vi "Affichage - 2 cam - 2P.vi"(8 "Couleur rectangle":u32(colorbox)=16775680, 9 "Caméra D":T1, 10 "Choix cam":u16, 11 "Caméra G":T1) -> (2 "Image 2D":picture)   [LabVIEW 2013]
uses:
  <vilib>/picture/picture.llb/Draw True-Color Pixmap.vi
panel:
  in  "Couleur rectangle 2":u32(colorbox)=16775680
  # "Affichage"
  # "Pour un rectangle"
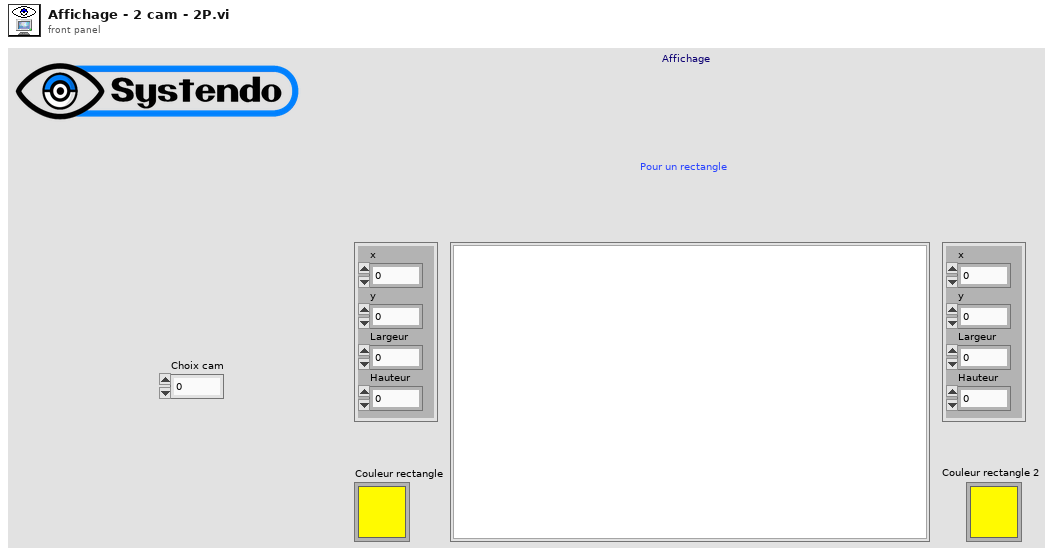
[diagram p1: front panel]
types:
  T1 = cluster{"x":i16, "y":i16, "Largeur":i16, "Hauteur":i16}
  T2 = typedef "imagedata.ctl" = cluster{"image type":i32, "image depth":i32, "image":u8[], "mask":u8[], "colors":u32[], "Rectangle":cluster{"left":i16, "top":i16, "right":i16, "bottom":i16}}
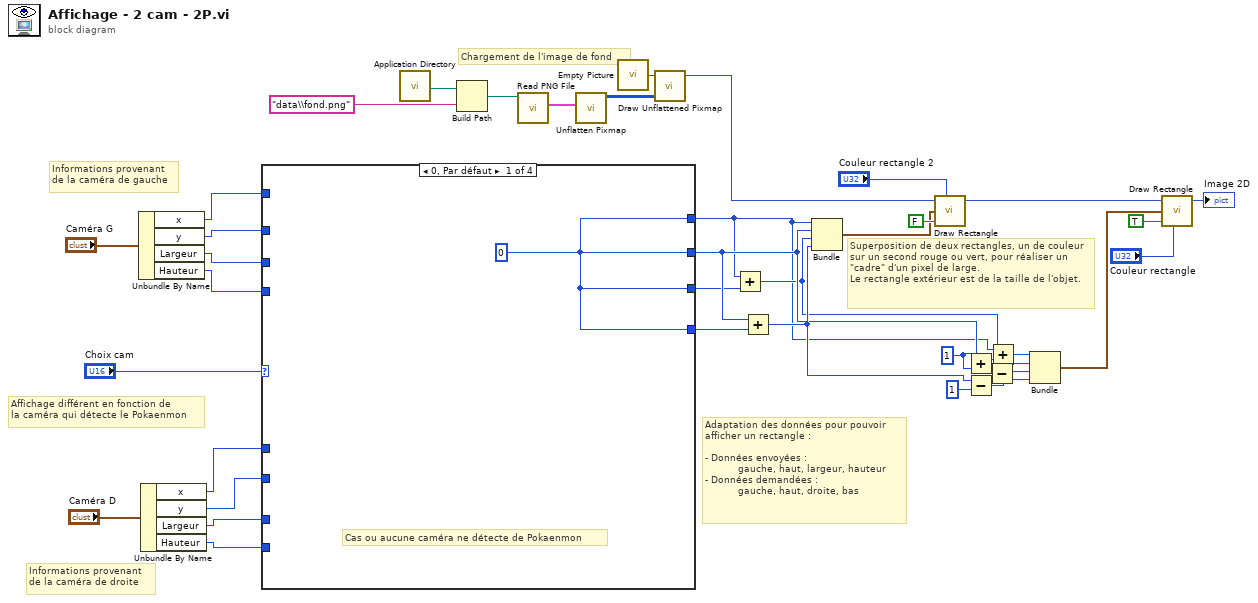
[diagram p0: block diagram]
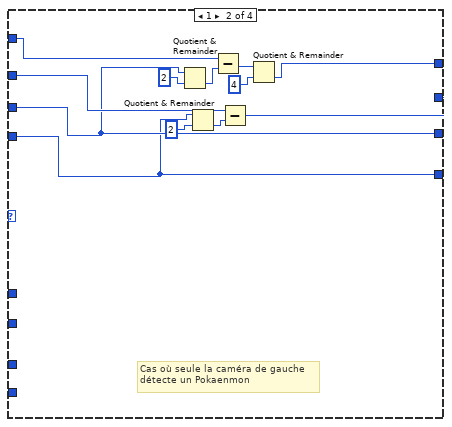
[diagram p2: hidden frame]
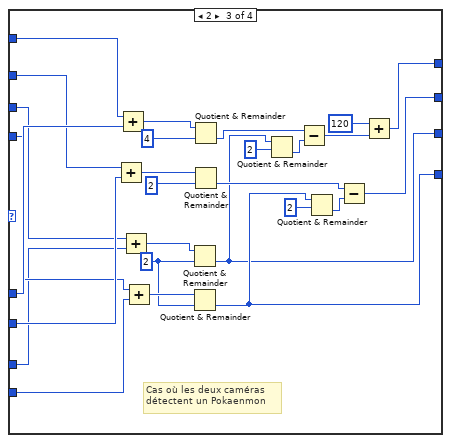
[diagram p3: hidden frame]
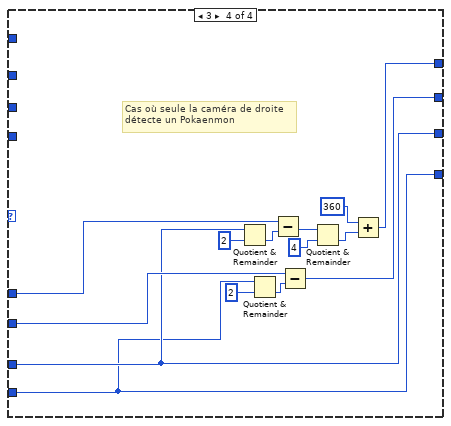
[diagram p4: hidden frame]
diagram:
  w15 = i16 1 ("y")
  w12 = i16 1 ("y")
  # "Chargement de l'image de fond"
  # "Superposition de deux rectangles, un de couleur sur un second rouge ou vert, pour réaliser un \"cadre\" d'un pixel de large.\nLe rectangle extérieur est de la taille de l'objet."
  # "Adaptation des données pour pouvoir\nafficher un rectangle :\n\n- Données envoyées :\n           gauche, haut, largeur, hauteur\n- Données demandées :\n           gauche, haut, droite, bas"
  # "Informations provenant\nde la caméra de droite"
  # "Informations provenant\nde la caméra de gauche"
  # "Affichage différent en fonction de\nla caméra qui détecte le Pokaenmon"
  n1 = Unbundle By Name("Caméra G") -> ("x"=w30:i16, "y"=w29:i16, "Largeur"=w28:i16, "Hauteur"=w27:i16)
  n2 = Unbundle By Name("Caméra D") -> ("x"=w23:i16, "y"=w24:i16, "Largeur"=w25:i16, "Hauteur"=w26:i16)
  n3 = case shown="0, Par défaut" "Choix cam" {
    tunnel: [w39 w43 w61 w88] -> w34
    tunnel: [w39 w49 w60 w90] -> w37
    tunnel: [w39 w47 w52 w83] -> w33
    tunnel: [w39 w41 w58 w80] -> w36
    tunnel: w23 -> [_ _ w71 w91]
    tunnel: w24 -> [_ _ w69 w92]
    tunnel: w25 -> [_ _ w66 w83]
    tunnel: w26 -> [_ _ w68 w80]
    tunnel: w27 -> [_ w41 w67 _]
    tunnel: w28 -> [_ w47 w65 _]
    tunnel: w29 -> [_ w50 w70 _]
    tunnel: w30 -> [_ w51 w72 _]
    frame 0, Default {
      w39 = 0
      # "Cas ou aucune caméra ne détecte de Pokaenmon"
    }
    frame 1 {
      # "Cas où seule la caméra de gauche\ndétecte un Pokaenmon"
      n4 = Quotient & Remainder(x=w47, y=u16 2) -> (floor(x/y)=w46:u16)  [unwired: 1 out]
      n5 = Quotient & Remainder(x=w41, y=u16 2) -> (floor(x/y)=w40:u16)  [unwired: 1 out]
      n6 = Subtract(x=w51, y=w46) -> (x-y=w44:u16)
      n7 = Subtract(x=w50, y=w40) -> (x-y=w49:u16)
      n8 = Quotient & Remainder(x=w44, y=u16 4) -> (floor(x/y)=w43:u16)  [unwired: 1 out]
    }
    frame 2 {
      w73 = i16 2 ("y")
      # "Cas où les deux caméras\ndétectent un Pokaenmon"
      n9 = Add(x=w70, y=w69) -> (x+y=w77:i16)
      n10 = Add(x=w72, y=w71) -> (x+y=w78:i16)
      n11 = Add(x=w65, y=w66) -> (x+y=w75:i16)
      n12 = Add(x=w67, y=w68) -> (x+y=w74:i16)
      n13 = Quotient & Remainder(x=w75, y=w73) -> (floor(x/y)=w52:i16)  [unwired: 1 out]
      n14 = Quotient & Remainder(x=w74, y=w73) -> (floor(x/y)=w58:i16)  [unwired: 1 out]
      n15 = Quotient & Remainder(x=w78, y=i16 4) -> (floor(x/y)=w54:i16)  [unwired: 1 out]
      n16 = Quotient & Remainder(x=w77, y=i16 2) -> (floor(x/y)=w63:i16)  [unwired: 1 out]
      n17 = Quotient & Remainder(x=w52, y=u16 2) -> (floor(x/y)=w55:u16)  [unwired: 1 out]
      n18 = Subtract(x=w54, y=w55) -> (x-y=w53:u16)
      n19 = Quotient & Remainder(x=w58, y=u16 2) -> (floor(x/y)=w57:u16)  [unwired: 1 out]
      n20 = Subtract(x=w63, y=w57) -> (x-y=w60:u16)
      n21 = Add(x=u16 120, y=w53) -> (x+y=w61:u16)
    }
    frame 3 {
      # "Cas où seule la caméra de droite\ndétecte un Pokaenmon"
      n22 = Quotient & Remainder(x=w83, y=u16 2) -> (floor(x/y)=w82:u16)  [unwired: 1 out]
      n23 = Quotient & Remainder(x=w80, y=u16 2) -> (floor(x/y)=w79:u16)  [unwired: 1 out]
      n24 = Subtract(x=w91, y=w82) -> (x-y=w86:u16)
      n25 = Subtract(x=w92, y=w79) -> (x-y=w90:u16)
      n26 = Quotient & Remainder(x=w86, y=u16 4) -> (floor(x/y)=w85:u16)  [unwired: 1 out]
      n27 = Add(x=u16 360, y=w85) -> (x+y=w88:u16)
    }
  }
  n28 = call <vilib>:"Application Directory.vi"() -> ("Application Directory"=w2:path)
  n29 = Build Path(base path=w2, name or relative path="data\\fond.png") -> (appended path=w3:path)
  n30 = call <vilib>:"Read PNG File.vi"("path to PNG file"=w3) -> ("image data"=w8:T2)  [unwired: 8 in, 2 out]
  n31 = call <vilib>:"Unflatten Pixmap.vi"("image data"=w8) -> ("24-bit pixmap"=w20:u32[][])  [unwired: 4 in, 6 out]
  n32 = call "Empty Picture"() -> ("empty picture"=w7:picture)
  n33 = call-poly <vilib>:"Draw Unflattened Pixmap.vi"("picture"=w7, "data (RGB format)"=w20) -> ("new picture"=w21:picture)  [unwired: 7 in]
  n34 = Add(x=w34, y=w33) -> (x+y=w35:i32)
  n35 = Add(x=w37, y=w36) -> (x+y=w38:i32)
  n36 = Bundle(w34, w37, w35, w38) -> (w5:cluster{i32, i32, i32, i32})  [unwired: 1 in]
  n37 = call <vilib>:"Draw Rectangle.vi"("picture"=w21, "rect"=w5, "fill?(F)"=FALSE, "color(black)"="Couleur rectangle 2") -> ("new picture"=w18:picture)  [unwired: 5 in]
  n38 = Add(x=w37, y=w12) -> (x+y=w11:i32)
  n39 = Subtract(x=w38, y=w15) -> (x-y=w14:i32)
  n40 = Subtract(x=w35, y=w15) -> (x-y=w13:i32)
  n41 = Add(x=w34, y=w12) -> (x+y=w10:i32)
  n42 = Bundle(w10, w11, w13, w14) -> (w16:cluster{i32, i32, i32, i32})  [unwired: 1 in]
  n43 = call <vilib>:"Draw Rectangle.vi"("picture"=w18, "rect"=w16, "fill?(F)"=TRUE, "color(black)"="Couleur rectangle") -> ("new picture"=→"Image 2D":picture)  [unwired: 5 in]
